vi "GenerateCommandString.vi"(0 "PC Status":i32=1, 1 "Port\nMotor":i32, 2 "Starboard\nMotor":i32, 3 "Left Rudder":i32, 4 "Right Rudder":i32, 5 "Pan Camera":i32(slide)=1500 scale=500.0..2500.0) -> (6 "CommandString":string)   [LabVIEW 2012]
doc: "Takes in speeds and/or directions for motors/servos and concatinates it into a command string to be sent over the XBee Radio to the Arbotix-M. To be used in tandum with the Xbaot_3.ios \n\nVictoria Coleman Feb 2013 (Adapted from Garland)"
panel:
  in  "String":string="$CS1500P1500R1500L1500P1500H   1\n"
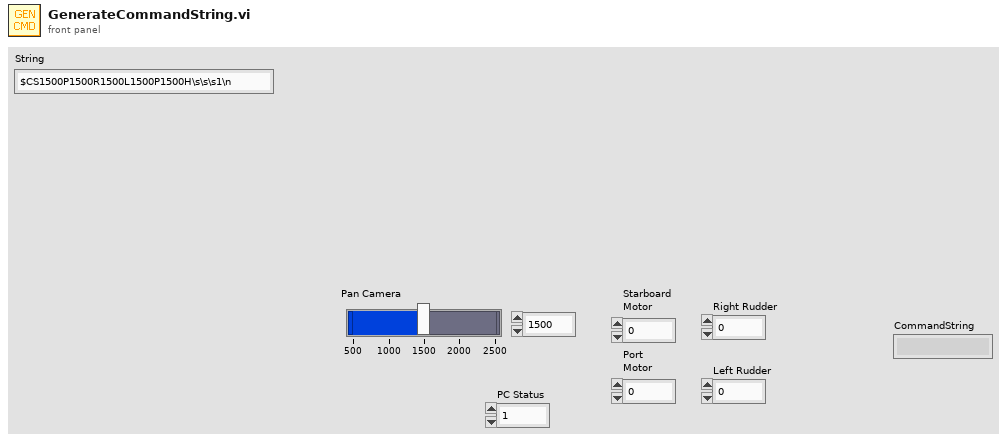
[diagram p1: front panel]
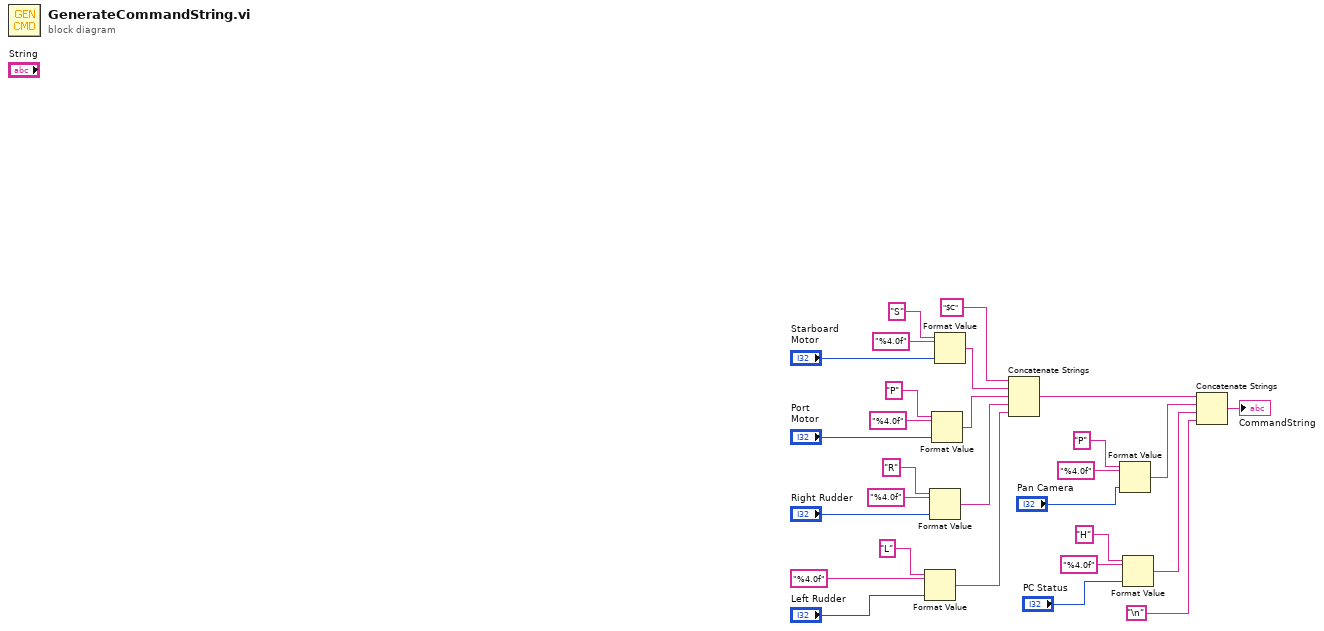
[diagram p0: block diagram]
diagram:
  n1 = Format Value(string ("")="L", format string="%4.0f", value (0)="Left Rudder") -> (output string=w16:string)
  n2 = Format Value(string ("")="R", format string="%4.0f", value (0)="Right Rudder") -> (output string=w17:string)
  n3 = Format Value(string ("")="P", format string="%4.0f", value (0)="Port\nMotor") -> (output string=w22:string)
  n4 = Format Value(string ("")="S", format string="%4.0f", value (0)="Starboard\nMotor") -> (output string=w23:string)
  n5 = Concatenate Strings("$C", w23, w22, w17, w16) -> (w11:string)
  n6 = Format Value(string ("")="P", format string="%4.0f", value (0)="Pan Camera") -> (output string=w10:string)
  n7 = Format Value(string ("")="H", format string="%4.0f", value (0)="PC Status") -> (output string=w9:string)
  n8 = Concatenate Strings(w11, w10, w9, "\n") -> (→"CommandString":string)
